vi "Global Debug Level.vi"() -> ()   [LabVIEW 2016, in "CS++Base.lvlib"]
uses:
  CS++Base.lvlib
  Severity.ctl
panel:
  in  "Debug Level":T1=enum."warning"
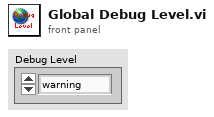
[diagram p1: front panel]
types:
  T1 = typedef "CS++Base.lvlib/Severity.ctl" = enum16{"emergency", "alert", "critical", "error", "warning", "notice", "info", "debug"}
diagram:
